vi "Create Temporary Transaction Table.vi"(8 "error in (no error)":errorcluster, 11 "Account History in":refnum<class "Account History.lvclass">) -> (0 "error out":errorcluster, 3 "Account History out":refnum<class "Account History.lvclass">)   [LabVIEW 2018, in "Account History.lvclass"]
uses:
  Account History.lvclass
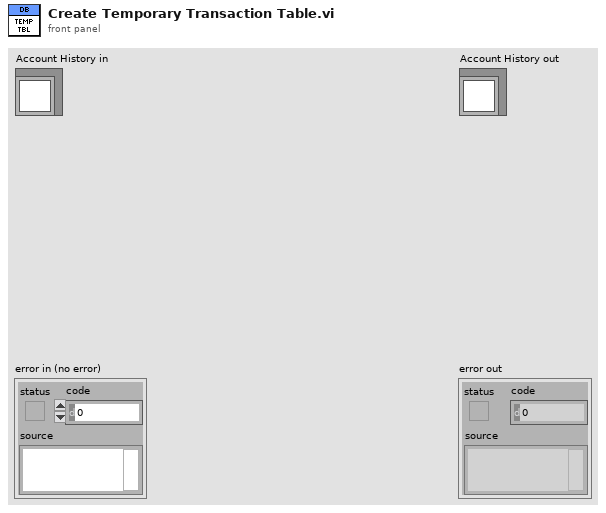
[diagram p1: front panel]
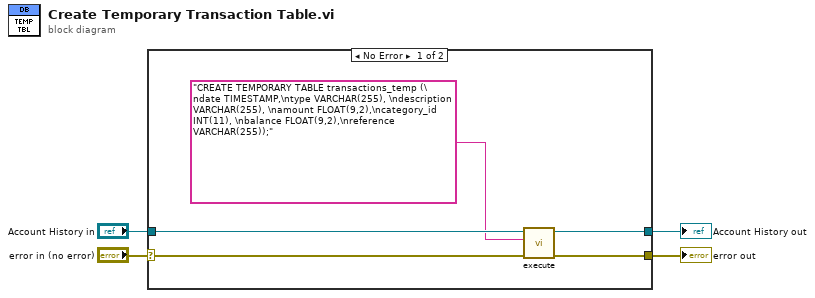
[diagram p0: block diagram]
diagram:
  n1 = case shown="No Error" "error in (no error)" {
    selector: "error in (no error)" -> [w7 w11]
    tunnel: [w6 w11] -> w3
    tunnel: [w8 w10] -> w1
    tunnel: "Account History in" -> [w9 w10]
    frame No Error {
      n2 = call "execute.vi"("error in (no error)"=w7, "SQL query"="CREATE TEMPORARY TABLE transactions_temp (\ndate TIMESTAMP,\ntype VARCHAR(255), \ndescription VARCHAR(255), \namount FLOAT(9,2),\ncategory_id INT(11), \nbalance FLOAT(9,2),\nreference VARCHAR(255));", "Database in"=w9) -> ("error out"=w6:errorcluster, "Database out"=w8:refnum<class "Account History.lvclass">)  [unwired: 7 in]
    }
    frame Error {
    }
  }
  "error out" <- w3
  "Account History out" <- w1
